vi "Periodic Tasks.vi"(8 "error in":errorcluster) -> ()   [LabVIEW 2020]
doc: "This VI runs in parallel to other tasks. It can contain as many user-defined periodic loops as you need. These can carry out PID or other sorts of timed response."
uses:
  <vilib>/Rock Robotics/WPI/Solenoid/WPI_SolenoidValue.ctl
  Robot Global Data.vi
  <vilib>/Rock Robotics/Network Tables/NT Write Number.vi
  <vilib>/addons/control/pid/pid.llb/PID (DBL).vi
  <vilib>/Rock Robotics/WPI/Solenoid/WPI_SolenoidSetEnum.vi
  <vilib>/Rock Robotics/WPI/Utilities/WPI_GetSetVariantRefNum.vi
  <vilib>/Rock Robotics/Network Tables/NT Write Variant.vi
  <vilib>/addons/control/pid/NI_PID_pid.lvlib
panel:
  out "error out":errorcluster
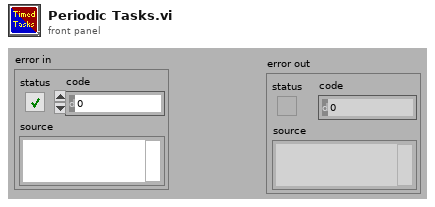
[diagram p1: front panel]
types:
  T1 = typedef "WPI_MotorControlDeviceRef.ctl" = cluster{"DeviceStatus":errorcluster, "Type":T2, "PWM":cluster{"PWM Channel":T3, "DeadBand":T4}, "CAN":cluster{"Device Number":u8, "SetOutput VI Ref":variant, "GetOutput VI Ref":variant, "Enable VI Ref":variant, "Disable VI Ref":variant, "Data":variant}, "Invert":bool, "DIO PWM":cluster{"PWM \"Enable\" Channel":T3, "DIOChannel":T5, "PWM Rate":dbl}}
  T2 = typedef "WPI_MotorControlType.ctl" = enum16{"PWM", "CAN", "DIO PWM"}
  T3 = typedef "FPGA_DIOPWMChannel.ctl" = enum8{"PWM 0", "PWM 1", "PWM 2", "PWM 3", "PWM 4", "PWM 5", "PWM 6", "PWM 7", "PWM 8", "PWM 9", "PWM MXP 0", "PWM MXP 1", "PWM MXP 2", "PWM MXP 3", "PWM MXP 4", "PWM MXP 5", "PWM MXP 6", "PWM MXP 7", "PWM MXP 8", "PWM MXP 9", "Invalid"}
  T4 = typedef "WPI_PWMDeadband.ctl" = cluster{"Name":string, "maxPositivePwm":i32, "minPositivePwm":i32, "centerPwm":i32, "maxNegativePwm":i32, "minNegativePwm":i32, "angularRange":u16}
  T5 = typedef "FPGA_DIOChannel.ctl" = enum8{"DIO 0", "DIO 1", "DIO 2", "DIO 3", "DIO 4", "DIO 5", "DIO 6", "DIO 7", "DIO 8", "DIO 9", "DIO MXP 0", "DIO MXP 1", "DIO MXP 2", "DIO MXP 3", "DIO MXP 4", "DIO MXP 5", "DIO MXP 6", "DIO MXP 7", "DIO MXP 8", "DIO MXP 9", "DIO MXP 10", "DIO MXP 11", "DIO MXP 12", "DIO MXP 13", "DIO MXP 14", "DIO MXP 15", "SPI Port CS1", "SPI Port CS2", "SPI Port CS3", "SPI Port MISO", "SPI Port MOSI", "Invalid"}
  T6 = typedef "FPGA_DutyCycleDevRef.ctl" = cluster{"DevStatus":errorcluster, "DutyCycleIndex":T7}
  T7 = typedef "FPGA_DutyCycleIndex.ctl" = enum8{"DutyCycle 0", "DutyCycle 1", "DutyCycle 2", "DutyCycle 3", "DutyCycle 4", "DutyCycle 5", "DutyCycle 6", "DutyCycle 7", "Invalid"}
  T8 = typedef "WPI_SolenoidDevRef.ctl" = cluster{"DevStatus":errorcluster, "Pneumatics Control Module":u8, "Forward Solenoid Channel":T9, "Reverse Solenoid Channel":T9}
  T9 = typedef "WPI_SolenoidChannel.ctl" = enum8{"Solenoid 0", "Solenoid 1", "Solenoid 2", "Solenoid 3", "Solenoid 4", "Solenoid 5", "Solenoid 6", "Solenoid 7", "Solenoid 8", "Solenoid 9", "Solenoid 10", "Solenoid 11", "Solenoid 12", "Solenoid 13", "Solenoid 14", "Solenoid 15", "Invalid"}
  T10 = typedef "ADIS16470 Device Reference.ctl" = cluster{"DevStatus":errorcluster, "Hardware Config":T11, "Calibration Complete":refnum<notifier>, "Status Reference":refnum<data-value>, "Data Reference":refnum<data-value>, "Sychronous Process VI":T14, "Cmd FIFO":refnum<k33>, "Source":T15, "Data FIFO":refnum<k33>, "Calibration Time (ms)":u32, "Data Reference":refnum<data-value>}
  T11 = typedef "ADIS16470 Hardware Configuration.ctl" = cluster{"SPI Clock Rate (Hz)":dbl, "IMU SPI Mode (3)":T12, "IMU Reset Pin":T5, "IMU SPI Bus":T13, "IMU Data Ready Pin":T5, "Stall Config":cluster{"Pow2BytesPerRead":u8, "StallTicks":u16, "CsToSclkTicks":u8}}
  T12 = typedef "WPI_SPIMode.ctl" = enum16{"Mode 0 (Clk Idle Low,Sample on Leading)", "Mode 1 (Clk Idle Low,Sample on Trailing)", "Mode 2 (Clk Idle High,Sample on Leading)", "Mode 3 (Clk Idle High,Sample on Trailing)"}
  T13 = typedef "spi_bus.ctl" = enum16{"SPI On-Board, CS0", "SPI On-Board, CS1", "SPI On-Board, CS2", "SPI On-Board, CS3", "SPI MXP", "Invalid"}
  T14 = typedef "ADIS16470 Process.ctl" = refnum<vi>
  T15 = typedef "FPGA_CounterEncoderSourceConvertionLVSourceType.ctl" = cluster{"DevStatus":errorcluster, "AnalogTriggerMode?":bool, "DigitalMode":cluster{"DIO Channel":T16}, "AnalogTriggerMode":cluster{"AnalogTriggerIndex":T17, "OutputType":T18}}
  T16 = typedef "FPGA_DIODigitalSourceChannel.ctl" = enum8{"DIO 0", "DIO 1", "DIO 2", "DIO 3", "DIO 4", "DIO 5", "DIO 6", "DIO 7", "DIO 8", "DIO 9", "DIO MXP 0", "DIO MXP 1", "DIO MXP 2", "DIO MXP 3", "DIO MXP 4", "DIO MXP 5", "DIO MXP 6", "DIO MXP 7", "DIO MXP 8", "DIO MXP 9", "DIO MXP 10", "DIO MXP 11", "DIO MXP 12", "DIO MXP 13", "DIO MXP 14", "DIO MXP 15", "SPI Port CS1", "SPI Port CS2", "SPI Port CS3", "SPI Port MISO", "SPI Port MOSI", "Disabled"}
  T17 = typedef "FPGA_AnalogTriggerIndex.ctl" = enum8{"Trig 0", "Trig 1", "Trig 2", "Trig 3", "Trig 4", "Trig 5", "Trig 6", "Trig 7", "Invalid"}
  T18 = typedef "FPGA_AnalogTriggerOutType.ctl" = enum16{"InWindow", "TriggerState", "Rising", "Falling"}
  T19 = typedef "WPI_JoystickDevRef.ctl" = cluster{"Device":T20}
  T20 = typedef "WPI_JoystickDeviceEnum.ctl" = enum16{"USB 0", "USB 1", "USB 2", "USB 3", "USB 4", "USB 5"}
  T21 = typedef "WPI_SolenoidValue.ctl" = enum16{"Off", "On", "Forward", "Reverse"}
  T22 = cluster{"proportional gain (Kc)":dbl, "integral time (Ti, min)":dbl, "derivative time (Td, min)":dbl}
  T23 = typedef "ADIS16470 Status.ctl" = cluster{"Calibrated?":bool, "IMU Detected?":bool}
  T24 = typedef "ADIS16470 Data.ctl" = cluster{"XAngle":dbl, "YAngle":dbl, "ZAngle":dbl}
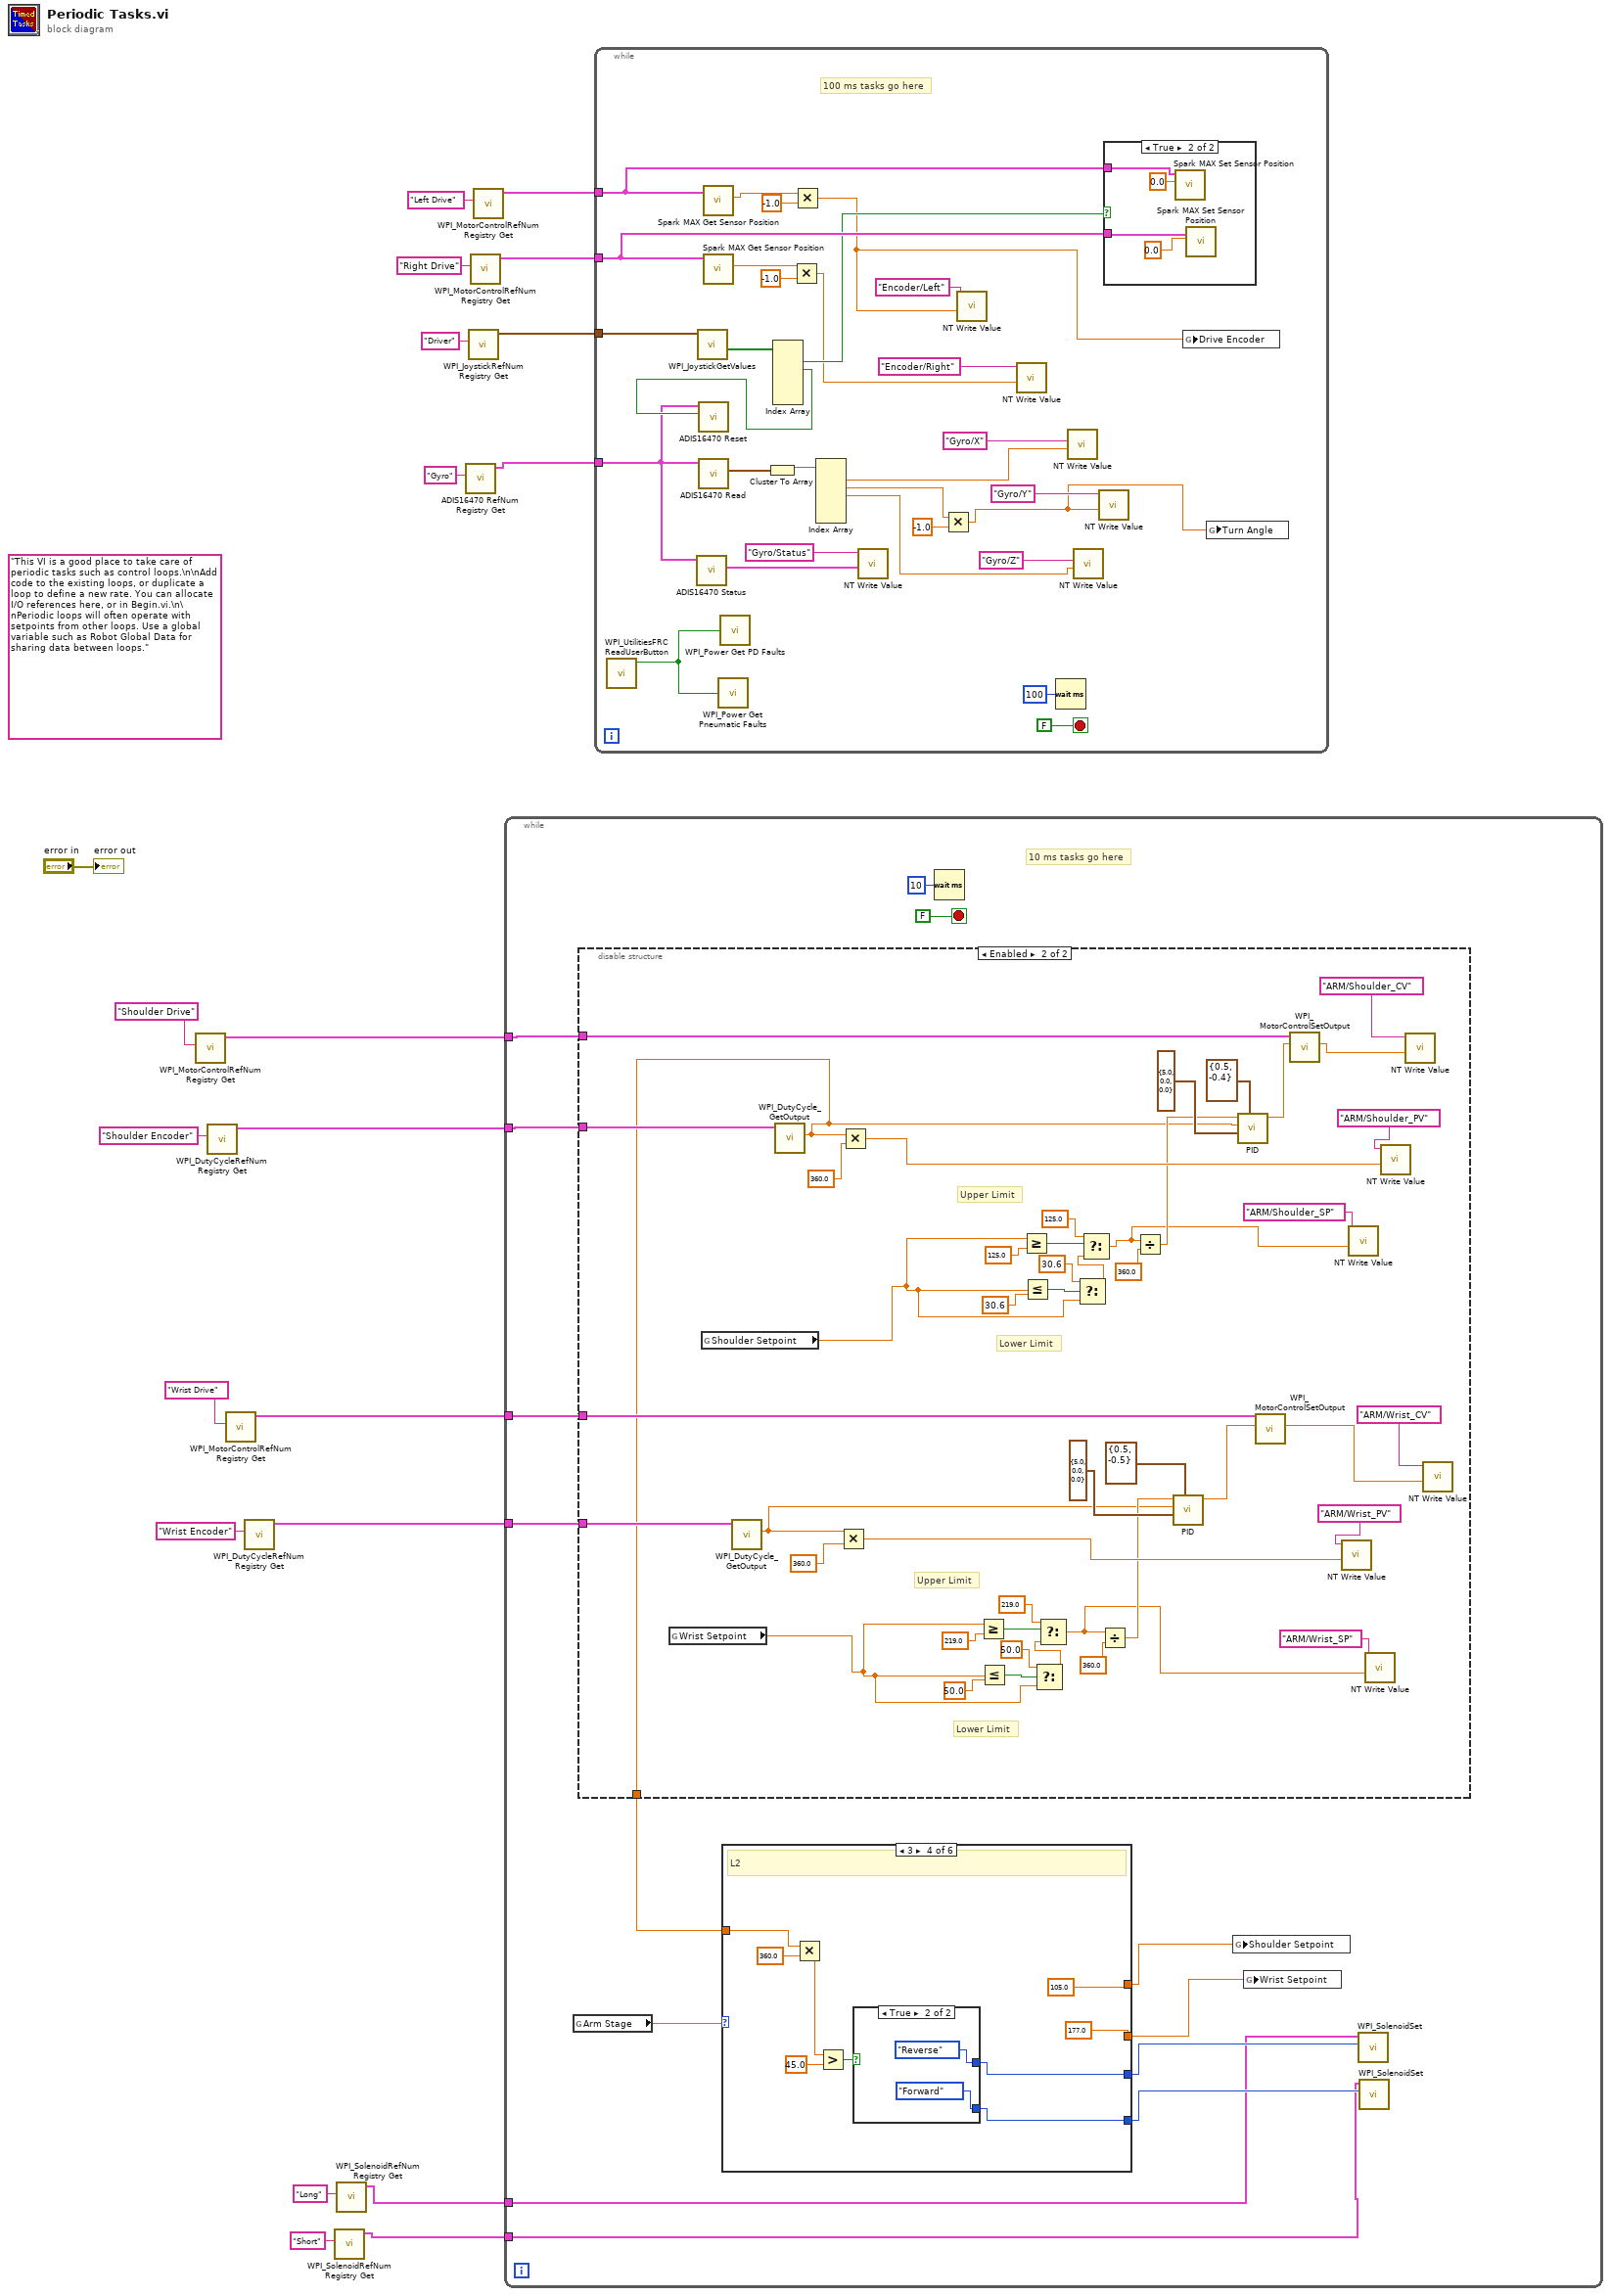
[diagram p0: block diagram]
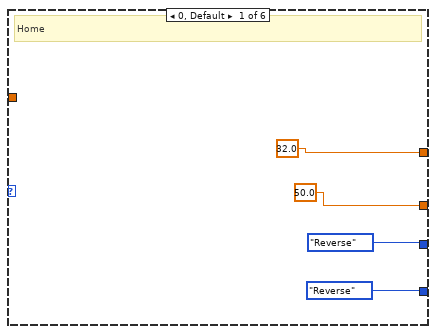
[diagram p2: hidden frame]
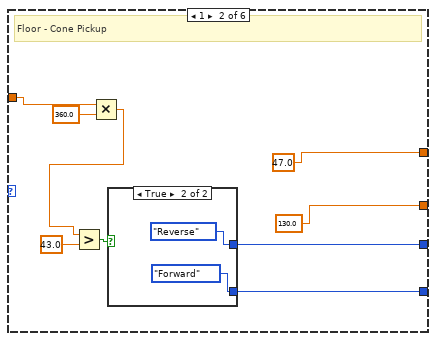
[diagram p3: hidden frame]
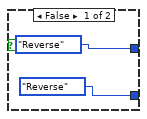
[diagram p4: hidden frame]
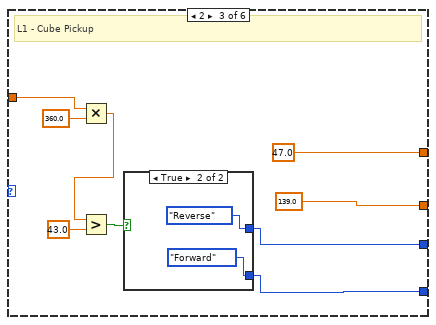
[diagram p5: hidden frame]
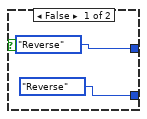
[diagram p6: hidden frame]
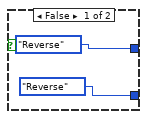
[diagram p7: hidden frame]
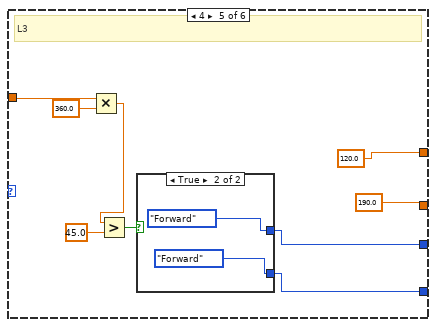
[diagram p8: hidden frame]
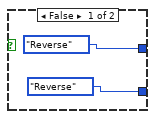
[diagram p9: hidden frame]
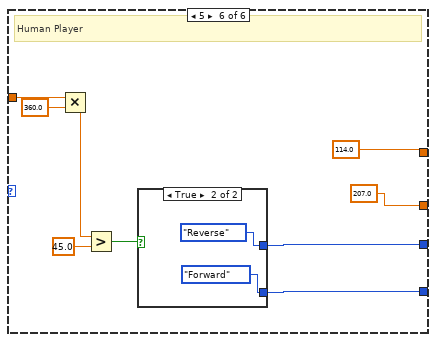
[diagram p10: hidden frame]
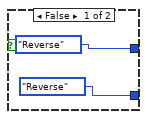
[diagram p11: hidden frame]
diagram:
  (unwired) "This VI is a good place to take care of periodic tasks such as control loops.\n\nAdd code to the existing loops, or duplicate a loop to define a new rate. You can allocate I/O references here, or in Begin.vi.\n\nPeriodic loops will often operate with setpoints from other loops. Use a global variable such as Robot Global Data for sharing data between loops."
  n1 = call <vilib>:"WPI_MotorControlRefNum Registry Get.vi"("refnum name"="Shoulder Drive") -> ("MotorControlDevRef"=w19:T1)  [unwired: 9 in, 1 out]
  n2 = call <vilib>:"WPI_DutyCycleRefNum Registry Get.vi"("refnum name"="Shoulder Encoder") -> ("DutyCycleDevRef"=w17:T6)  [unwired: 9 in, 1 out]
  n3 = call <vilib>:"WPI_MotorControlRefNum Registry Get.vi"("refnum name"="Wrist Drive") -> ("MotorControlDevRef"=w13:T1)  [unwired: 9 in, 1 out]
  n4 = call <vilib>:"WPI_DutyCycleRefNum Registry Get.vi"("refnum name"="Wrist Encoder") -> ("DutyCycleDevRef"=w15:T6)  [unwired: 9 in, 1 out]
  n5 = call <vilib>:"WPI_SolenoidRefNum Registry Get.vi"("refnum name"="Short") -> ("SolenoidDevRef"=w9:T8)  [unwired: 9 in, 1 out]
  n6 = call <vilib>:"WPI_SolenoidRefNum Registry Get.vi"("refnum name"="Long") -> ("SolenoidDevRef"=w10:T8)  [unwired: 9 in, 1 out]
  n7 = call <vilib>:"ADIS16470 RefNum Registry Get.vi"("refnum name"="Gyro") -> ("ADIS16470DevRef out"=w2:T10)  [unwired: 9 in, 1 out]
  n8 = call <vilib>:"WPI_JoystickRefNum Registry Get.vi"("refnum name"="Driver") -> ("JoystickDevRef"=w3:T19)  [unwired: 9 in, 1 out]
  n9 = call <vilib>:"WPI_MotorControlRefNum Registry Get.vi"("refnum name"="Right Drive") -> ("MotorControlDevRef"=w7:T1)  [unwired: 9 in, 1 out]
  n10 = call <vilib>:"WPI_MotorControlRefNum Registry Get.vi"("refnum name"="Left Drive") -> ("MotorControlDevRef"=w8:T1)  [unwired: 9 in, 1 out]
  n11 = while {
    tunnel: w19 -> [w31]
    tunnel: w17 -> [w30]
    tunnel: w15 -> [w32]
    tunnel: w13 -> [w33]
    tunnel: w10 -> [w26]
    tunnel: w9 -> [w25]
    stop <- FALSE stop-if-true
    # "10 ms tasks go here"
    n12 = global read "Robot Global Data.vi" "Arm Stage"() -> (w22:dbl)
    n13 = disable-structure shown="Enabled" {
      disable-tunnel: w33 -> [_ w135]
      disable-tunnel: w32 -> [_ w134]
      disable-tunnel: w31 -> [_ w118]
      disable-tunnel: w30 -> [_ w114]
      disable-tunnel: [_ w105] -> w29
      frame Disabled {
      }
      frame Enabled {
        # "Lower Limit"
        # "Upper Limit"
        # "Lower Limit"
        # "Upper Limit"
        n14 = global read "Robot Global Data.vi" "Wrist Setpoint"() -> (w150:dbl)
        n15 = global read "Robot Global Data.vi" "Shoulder Setpoint"() -> (w131:dbl)
        n16 = call <vilib>:"WPI_DutyCycle_GetOutput.vi"("DutyCycleDevRef"=w134) -> ("Output"=w108:dbl)  [unwired: 8 in, 2 out]
        n17 = call <vilib>:"WPI_DutyCycle_GetOutput.vi"("DutyCycleDevRef"=w114) -> ("Output"=w105:dbl)  [unwired: 8 in, 2 out]
        n18 = Multiply(x=w108, y=360.0) -> (x*y=w149:dbl)
        n19 = Multiply(x=w105, y=360.0) -> (x*y=w130:dbl)
        n20 = Greater Or Equal?(x=w150, y=219.0) -> (x >= y?=w147:bool)
        n21 = Less Or Equal?(x=w150, y=50.0) -> (x <= y?=w148:bool)
        n22 = Greater Or Equal?(x=w131, y=125.0) -> (x >= y?=w128:bool)
        n23 = Less Or Equal?(x=w131, y=30.6) -> (x <= y?=w129:bool)
        n24 = Select(t=50.0, s=w148, f=w150) -> (s? t:f=w146:dbl)
        n25 = Select(t=219.0, s=w147, f=w146) -> (s? t:f=w106:dbl)
        n26 = Select(t=30.6, s=w129, f=w131) -> (s? t:f=w127:dbl)
        n27 = Select(t=125.0, s=w128, f=w127) -> (s? t:f=w107:dbl)
        n28 = Divide(x=w106, y=360.0) -> (x/y=w109:dbl)
        n29 = Divide(x=w107, y=360.0) -> (x/y=w112:dbl)
        n30 = call-poly <vilib>:"PID.vi"("output range"=cluster{"output high":dbl, "output low":dbl} {"output high"=0.5, "output low"=-0.5}, "PID gains"=T22 {"proportional gain (Kc)"=5.0, "integral time (Ti, min)"=0.0, "derivative time (Td, min)"=0.0}, "process variable"=w108, "setpoint"=w109) -> ("output"=w144:dbl)  [unwired: 6 in, 1 out]
        n31 = call-poly <vilib>:"PID.vi"("output range"=cluster{"output high":dbl, "output low":dbl} {"output high"=0.5, "output low"=-0.4}, "PID gains"=T22 {"proportional gain (Kc)"=5.0, "integral time (Ti, min)"=0.0, "derivative time (Td, min)"=0.0}, "process variable"=w105, "setpoint"=w112) -> ("output"=w125:dbl)  [unwired: 6 in, 1 out]
        n32 = call <vilib>:"WPI_MotorControlSetOutput.vi"("Output"=w144, "MotorControlDevRef"=w135) -> ("Motor Output"=w145:dbl)  [unwired: 7 in, 2 out]
        n33 = call <vilib>:"WPI_MotorControlSetOutput.vi"("Output"=w125, "MotorControlDevRef"=w118) -> ("Motor Output"=w126:dbl)  [unwired: 7 in, 2 out]
        n34 = call-poly <vilib>:"NT Write Value.vi"("value"=w149, "name"="ARM/Wrist_PV") -> ()  [unwired: 9 in, 1 out]
        n35 = call-poly <vilib>:"NT Write Value.vi"("value"=w107, "name"="ARM/Shoulder_SP") -> ()  [unwired: 9 in, 1 out]
        n36 = call-poly <vilib>:"NT Write Value.vi"("value"=w106, "name"="ARM/Wrist_SP") -> ()  [unwired: 9 in, 1 out]
        n37 = call-poly <vilib>:"NT Write Value.vi"("value"=w130, "name"="ARM/Shoulder_PV") -> ()  [unwired: 9 in, 1 out]
        n38 = call-poly <vilib>:"NT Write Value.vi"("value"=w126, "name"="ARM/Shoulder_CV") -> ()  [unwired: 9 in, 1 out]
        n39 = call-poly <vilib>:"NT Write Value.vi"("value"=w145, "name"="ARM/Wrist_CV") -> ()  [unwired: 9 in, 1 out]
      }
    }
    n40 = case "Setpoints for Arm" shown="3" w22 {
      tunnel: [50.0 ("t") 130.0 ("t") 139.0 ("t") 177.0 ("t") 190.0 ("t") 207.0 ("t")] -> w23
      tunnel: [32.0 ("t") 47.0 ("t") 47.0 ("t") 105.0 ("t") 120.0 ("t") 114.0 ("t")] -> w24
      tunnel: [WPI_SolenoidValue."Reverse" ("Value") w45 w58 w71 w84 w97] -> w28
      tunnel: [WPI_SolenoidValue."Reverse" ("Value") w44 w57 w70 w83 w96] -> w27
      tunnel: w29 -> [_ w41 w54 w67 w80 w94]
      frame 0, Default {
        # "Home"
      }
      frame 1 {
        # "Floor - Cone Pickup"
        n41 = Multiply(x=w41, y=360.0) -> (x*y=w40:dbl)
        n42 = Greater?(x=w40, y=43.0) -> (0:w43:bool)
        n43 = case shown="True" w43 {
          tunnel: [WPI_SolenoidValue."Reverse" ("Value") WPI_SolenoidValue."Reverse" ("Value")] -> w45
          tunnel: [WPI_SolenoidValue."Reverse" ("Value") WPI_SolenoidValue."Forward" ("Value")] -> w44
          frame False {
          }
          frame True {
          }
        }
      }
      frame 2 {
        # "L1 - Cube Pickup"
        n44 = Multiply(x=w54, y=360.0) -> (x*y=w53:dbl)
        n45 = Greater?(x=w53, y=43.0) -> (0:w56:bool)
        n46 = case shown="True" w56 {
          tunnel: [WPI_SolenoidValue."Reverse" ("Value") WPI_SolenoidValue."Reverse" ("Value")] -> w58
          tunnel: [WPI_SolenoidValue."Reverse" ("Value") WPI_SolenoidValue."Forward" ("Value")] -> w57
          frame False {
          }
          frame True {
          }
        }
      }
      frame 3 {
        # "L2"
        n47 = Multiply(x=w67, y=360.0) -> (x*y=w66:dbl)
        n48 = Greater?(x=w66, y=45.0) -> (0:w69:bool)
        n49 = case shown="True" w69 {
          tunnel: [WPI_SolenoidValue."Reverse" ("Value") WPI_SolenoidValue."Reverse" ("Value")] -> w71
          tunnel: [WPI_SolenoidValue."Reverse" ("Value") WPI_SolenoidValue."Forward" ("Value")] -> w70
          frame False {
          }
          frame True {
          }
        }
      }
      frame 4 {
        # "L3"
        n50 = Multiply(x=w80, y=360.0) -> (x*y=w79:dbl)
        n51 = Greater?(x=w79, y=45.0) -> (0:w82:bool)
        n52 = case shown="True" w82 {
          tunnel: [WPI_SolenoidValue."Reverse" ("Value") WPI_SolenoidValue."Forward" ("Value")] -> w84
          tunnel: [WPI_SolenoidValue."Reverse" ("Value") WPI_SolenoidValue."Forward" ("Value")] -> w83
          frame False {
          }
          frame True {
          }
        }
      }
      frame 5 {
        # "Human Player"
        n53 = Multiply(x=w94, y=360.0) -> (x*y=w92:dbl)
        n54 = Greater?(x=w92, y=45.0) -> (0:w95:bool)
        n55 = case shown="True" w95 {
          tunnel: [WPI_SolenoidValue."Reverse" ("Value") WPI_SolenoidValue."Reverse" ("Value")] -> w97
          tunnel: [WPI_SolenoidValue."Reverse" ("Value") WPI_SolenoidValue."Forward" ("Value")] -> w96
          frame False {
          }
          frame True {
          }
        }
      }
    }
    n56 = Wait (ms)(milliseconds to wait=u32 10) -> ()  [unwired: 1 out]
    n57 = global write "Robot Global Data.vi" "Shoulder Setpoint"(w24) -> ()
    n58 = global write "Robot Global Data.vi" "Wrist Setpoint"(w23) -> ()
    n59 = call-poly <vilib>:"WPI_SolenoidSet.vi"("Value"=w28, "SolenoidDevRef"=w26) -> ()  [unwired: 8 in, 2 out]
    n60 = call-poly <vilib>:"WPI_SolenoidSet.vi"("Value"=w27, "SolenoidDevRef"=w25) -> ()  [unwired: 8 in, 2 out]
  }
  n61 = while {
    tunnel: w8 -> [w177]
    tunnel: w7 -> [w176]
    tunnel: w3 -> [w175]
    tunnel: w2 -> [w171]
    stop <- FALSE stop-if-true
    # "100 ms tasks go here"
    n62 = call <vilib>:"WPI_UtilitiesFRC ReadUserButton.vi"() -> ("User Button"=w178:bool)  [unwired: 10 in, 1 out]
    n63 = call <vilib>:"ADIS16470 Status.vi"("ADIS16470DevRef"=w171) -> ("ADIS16470 Status"=w170:T23)  [unwired: 8 in, 2 out]
    n64 = call <vilib>:"WPI_JoystickGetValues.vi"("JoystickDevRef"=w175) -> ("Buttons"=w174:bool[])  [unwired: 6 in, 4 out]
    n65 = call <vilib>:"ADIS16470 Read.vi"("ADIS16470DevRef"=w171) -> ("ADIS16470 Value"=w165:T24)  [unwired: 7 in, 3 out]
    n66 = call <vilib>:"Spark MAX Get Sensor Position.vi"("MotorControlDevRef in"=w177) -> ("Sensor Position"=w155:dbl)  [unwired: 7 in, 3 out]
    n67 = call <vilib>:"Spark MAX Get Sensor Position.vi"("MotorControlDevRef in"=w176) -> ("Sensor Position"=w154:dbl)  [unwired: 7 in, 3 out]
    n68 = call <vilib>:"WPI_Power Get Pneumatic Faults.vi"("Clear Sticky Faults"=w178) -> ()  [unwired: 9 in, 6 out]
    n69 = call <vilib>:"WPI_Power Get PD Faults.vi"("Clear Sticky Faults"=w178) -> ()  [unwired: 11 in, 4 out]
    n70 = Cluster To Array(cluster=w165) -> (array=w164:dbl[])
    n71 = Index Array(array=w174) -> (element #1=w173:bool, element #2=w172:bool)  [unwired: 6 in, 4 out]
    n72 = call <vilib>:"ADIS16470 Reset.vi"("Reset? (T)"=w172, "ADIS16470DevRef"=w171) -> ()  [unwired: 8 in, 2 out]
    n73 = Multiply(x=w154, y=-1.0) -> (x*y=w156:dbl)
    n74 = Multiply(x=w155, y=-1.0) -> (x*y=w151:dbl)
    n75 = Index Array(array=w164) -> (element #1=w161:dbl, element #2=w159:dbl, element #3=w160:dbl)  [unwired: 6 in, 3 out]
    n76 = call-poly <vilib>:"NT Write Value.vi"("variant"=w170, "name"="Gyro/Status") -> ()  [unwired: 9 in, 1 out]
    n77 = Multiply(x=w159, y=-1.0) -> (x*y=w157:dbl)
    n78 = call-poly <vilib>:"NT Write Value.vi"("value"=w151, "name"="Encoder/Left") -> ()  [unwired: 9 in, 1 out]
    n79 = call-poly <vilib>:"NT Write Value.vi"("value"=w156, "name"="Encoder/Right") -> ()  [unwired: 9 in, 1 out]
    n80 = Wait (ms)(milliseconds to wait=u32 100) -> ()  [unwired: 1 out]
    n81 = call-poly <vilib>:"NT Write Value.vi"("value"=w161, "name"="Gyro/X") -> ()  [unwired: 9 in, 1 out]
    n82 = call-poly <vilib>:"NT Write Value.vi"("value"=w160, "name"="Gyro/Z") -> ()  [unwired: 9 in, 1 out]
    n83 = call-poly <vilib>:"NT Write Value.vi"("value"=w157, "name"="Gyro/Y") -> ()  [unwired: 9 in, 1 out]
    n84 = case shown="True" w173 {
      tunnel: w177 -> [_ w183]
      tunnel: w176 -> [_ w181]
      frame False {
      }
      frame True {
        n85 = call <vilib>:"Spark MAX Set Sensor Position.vi"("Position"=0.0, "MotorControlDeviceRef"=w183) -> ()  [unwired: 8 in, 2 out]
        n86 = call <vilib>:"Spark MAX Set Sensor Position.vi"("Position"=0.0, "MotorControlDeviceRef"=w181) -> ()  [unwired: 8 in, 2 out]
      }
    }
    n87 = global write "Robot Global Data.vi" "Drive Encoder"(w151) -> ()
    n88 = global write "Robot Global Data.vi" "Turn Angle"(w157) -> ()
  }
  "error out" <- "error in"
